vi "Select Object.vi"(10 "Coords":T5, 11 "Core Data in":T3) -> (1 "Diffuse Colour":u32(colorbox), 2 "Transform":T1, 3 "Core Data out":T3)   [LabVIEW 2022 SP3, in "Application.lvlib"]
uses:
  Application.lvlib
  <vilib>/Utility/miscctls.llb/LVPoint32TypeDef.ctl
  Core Data.ctl
  Scene/Scene.lvclass
  Libraries/3D/Transform.ctl
  Libraries/3D/Vector 3D.ctl
  Mouse Button Held.ctl
  Libraries/3D/3D.lvlib
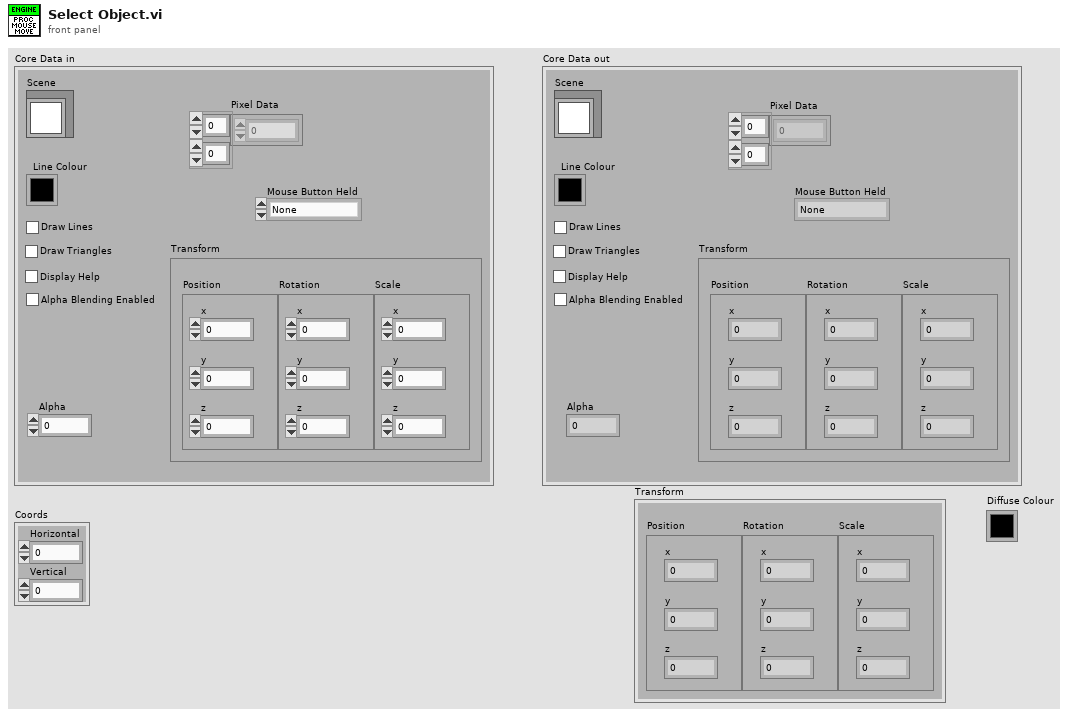
[diagram p1: front panel]
types:
  T1 = typedef "3D.lvlib/Transform.ctl" = cluster{"Position":T2, "Rotation":T2, "Scale":T2}
  T2 = typedef "3D.lvlib/Vector 3D.ctl" = cluster{"x":sgl, "y":sgl, "z":sgl}
  T3 = typedef "Application.lvlib/Core Data.ctl" = cluster{"Line Colour":u32, "Draw Lines":bool, "Draw Triangles":bool, "Pixel Data":u32[][], "Scene":refnum<class "Scene.lvclass">, "Display Help":bool, "Transform":T1, "Alpha":dbl, "Mouse Button Held":T4, "Alpha Blending Enabled":bool}
  T4 = typedef "Application.lvlib/Mouse Button Held.ctl" = enum16{"None", "Left", "Middle", "Right"}
  T5 = typedef "LVPoint32TypeDef.ctl" = cluster{"Horizontal":i32, "Vertical":i32}
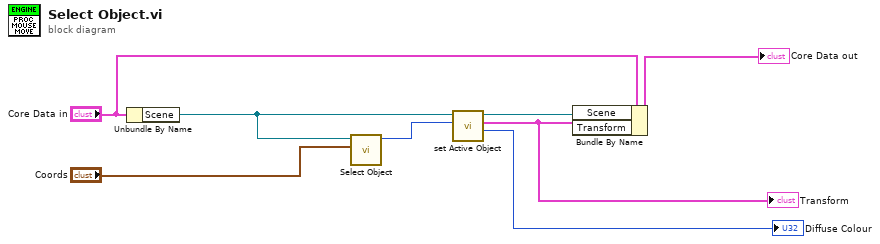
[diagram p0: block diagram]
diagram:
  n1 = Unbundle By Name("Core Data in") -> ("Scene"=w4:refnum<class "Scene.lvclass">)
  n2 = call "Select Object.vi"("Coords"="Coords", "Scene in"=w4) -> ("Active Object"=w3:i32)  [unwired: 9 in]
  n3 = call "set Active Object.vi"("Active Object"=w3, "Scene in"=w4) -> ("Diffuse Colour"=→"Diffuse Colour":u32, "Transform"=w2:T1, "Scene out"=w5:refnum<class "Scene.lvclass">)  [unwired: 7 in]
  "Transform" <- w2
  n4 = Bundle By Name(cluster="Core Data in", "Scene"=w5, "Transform"=w2) -> (→"Core Data out":T3)
